vi "Pressure Sensor (Read).vi"(6 "ISOBUS address":T3=-1 caption="ISOBUS address (-1)", 8 "error in":errorcluster, 11 "Mercury Reference In":T4) -> (0 "error out":errorcluster, 2 "Sensor Type":T2, 3 "Mercury Reference Out":T4, 4 "Valid?":T1)   [LabVIEW 2015, in "Mercury iXX.lvlib" / "Pressure.lvlib"]
doc: "Read the sensor type of the selected pressure device."
uses:
  Pressure.lvlib
  Controls/Mercury Reference.ctl
  Controls/Comms Transport Layer.ctl
  private/Controls/Query Dynamic Reference.ctl
  Controls/ISOBus Address.ctl
  Controls/Pressure Sensor Type.ctl
  Controls/Is Valid LED.ctl
  private/Controls/Command Verbs.ctl
  Mercury iXX.lvlib
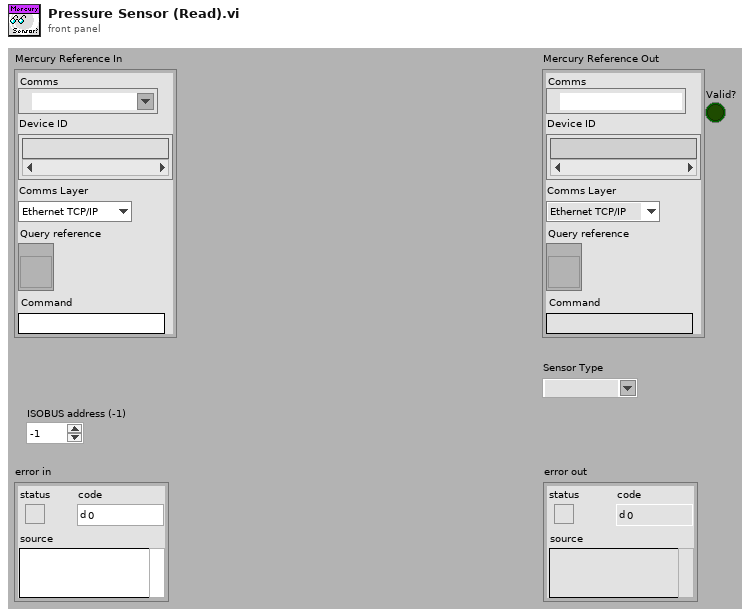
[diagram p1: front panel]
types:
  T1 = typedef "Mercury iXX.lvlib/Is Valid LED.ctl" = bool
  T2 = typedef "Mercury iXX.lvlib/Pressure.lvlib/Pressure Sensor Type.ctl" = string
  T3 = typedef "Mercury iXX.lvlib/ISOBus Address.ctl" = i32
  T4 = typedef "Mercury iXX.lvlib/Mercury Reference.ctl" = cluster{"Comms":refnum<visa-resource-name>, "Device ID":string[], "Comms Layer":T5, "Command":string, "Query reference":T6}
  T5 = typedef "Mercury iXX.lvlib/Comms Transport Layer.ctl" = enum16{"Ethernet TCP/IP", "USB", "ISOBus - RS-232", "GPIB"}
  T6 = typedef "Mercury iXX.lvlib/Query Dynamic Reference.ctl" = refnum<vi>
  T7 = typedef "Mercury iXX.lvlib/Command Verbs.ctl" = string
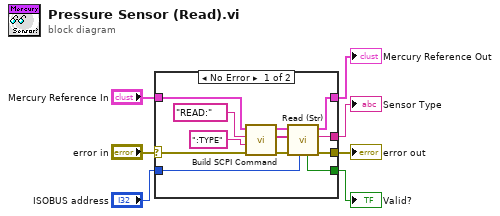
[diagram p0: block diagram]
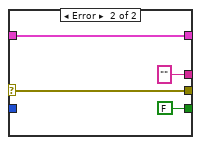
[diagram p2: hidden frame]
diagram:
  n1 = case shown="No Error" "error in" {
    selector: "error in" -> [w8 w23]
    tunnel: "Mercury Reference In" -> [w14 w22]
    tunnel: [w13 w22] -> w6
    tunnel: [w12 w23] -> w5
    tunnel: "ISOBUS address" -> [w11 _]
    tunnel: [w10 T1 FALSE ("Valid?")] -> w3
    tunnel: [w9 "" ("Response")] -> w2
    frame No Error {
      n2 = call "Build SCPI Command.vi"("error in"=w8, "Noun(s)"=":TYPE" ("Command"), "Verb"=T7 "READ:", "Mercury Reference In"=w14) -> ("error out"=w19:errorcluster, "SCPI Message(s)"=w16:string[], "Mercury Reference Out"=w17:T4)  [unwired: 5 out]
      n3 = call "Read (Str).vi"("ISOBUS address"=w11, "error in"=w19, "SCPI Message(s)"=w16, "Mercury Reference In"=w17) -> ("error out"=w12:errorcluster, "Response"=w9:string, "Mercury Reference Out"=w13:T4, "Valid?"=w10:T1)  [unwired: 4 out]
    }
    frame Error {
    }
  }
  "Mercury Reference Out" <- w6
  "error out" <- w5
  "Sensor Type" <- w2
  "Valid?" <- w3
